vi "getMessage.vi"(8 "error in (no error)":errorcluster, 11 "PriorityNode in":refnum<class "PriorityNode.lvclass">) -> (0 "error out":errorcluster, 2 "Message.lvclass":refnum<class "Message.lvclass">, 3 "PriorityNode out":refnum<class "PriorityNode.lvclass">)   [LabVIEW 2009, in "PriorityNode.lvclass"]
uses:
  PriorityNode.lvclass
  Message/Message.lvclass
  PriorityNode.lvclass/PriorityNode.ctl
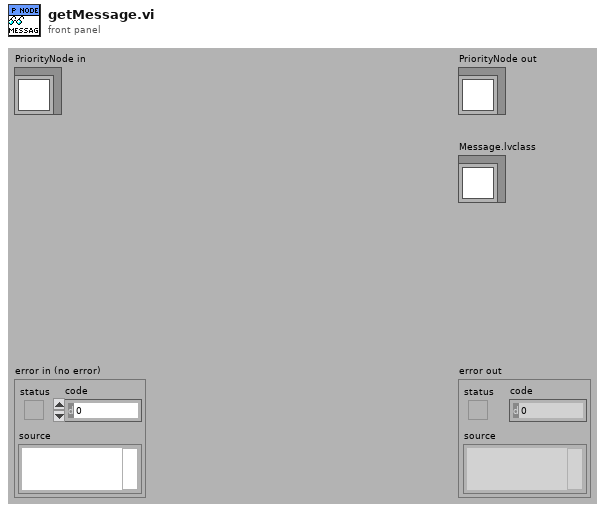
[diagram p1: front panel]
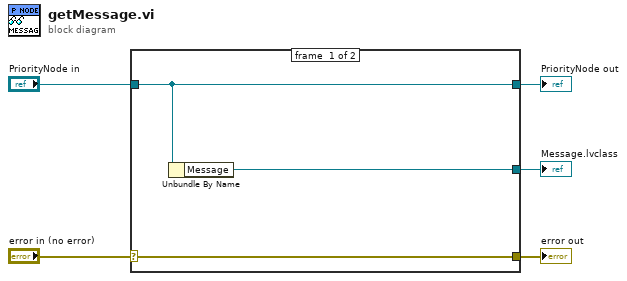
[diagram p0: block diagram]
diagram:
  n1 = case shown="No Error" "error in (no error)" {
    selector: "error in (no error)" -> [w8 w9]
    tunnel: [w8 w9] -> w4
    tunnel: [w7 w10] -> w2
    tunnel: "PriorityNode in" -> [w7 w10]
    tunnel: [w6 _] -> w1
    frame #0 {
      n2 = Unbundle By Name(w7) -> ("Message"=w6:refnum<class "Message.lvclass">)
    }
    frame #1 {
    }
  }
  "error out" <- w4
  "PriorityNode out" <- w2
  "Message.lvclass" <- w1
